vi "Status Display.vi"(6 "Action":enum16{"Update", "Clear"}(ring), 8 "error in":errorcluster, 11 "Status line":string) -> (0 "error out":errorcluster, 3 "Status":string)   [LabVIEW 2016]
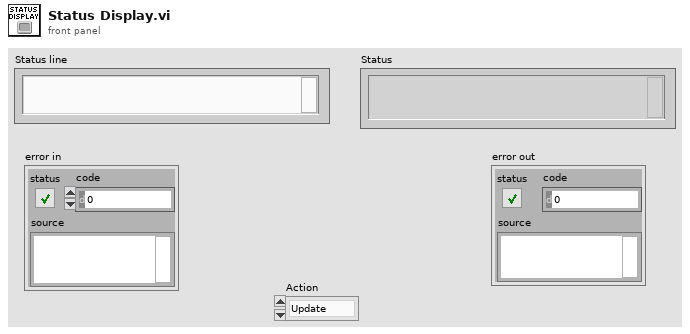
[diagram p1: front panel]
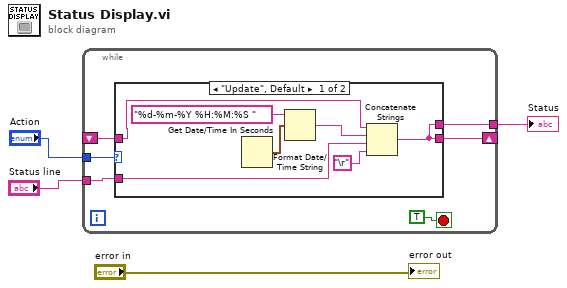
[diagram p0: block diagram]
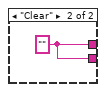
[diagram p2: hidden frame]
diagram:
  n1 = while {
    tunnel: "Action" -> [w9]
    tunnel: "Status line" -> [w8]
    tunnel: [w7] -> w4
    shift-right: [w6] -> _
    shift-left: _ -> [w5]
    stop <- TRUE stop-if-true
    n2 = case shown="\"Update\", Default" w9 {
      tunnel: w8 -> [w13 _]
      tunnel: [w12 w18] -> w7
      tunnel: [w12 w18] -> w6
      tunnel: w5 -> [w11 _]
      frame "Update", Default {
        n3 = Get Date/Time In Seconds() -> (seconds since 1Jan1904=w14:timestamp)
        n4 = Format Date/Time String(time format string (%c)="%d-%m-%Y %H:%M:%S ", seconds (now)=w14) -> (date/time string=w16:string)  [unwired: 1 in]
        n5 = Concatenate Strings(w11, w16, w13, "\r") -> (w12:string)
      }
      frame "Clear" {
        w18 = "" ("Status")
      }
    }
  }
  "Status" <- w4
  "error out" <- "error in"
